vi "FilterPointNameToFloat.vi"(11 "RobotPoints in":string[][](array[string])) -> (0 "U":dbl, 1 "Z":dbl, 2 "V":dbl, 3 "Hand":string, 4 "Y":dbl, 5 "W":dbl, 6 "X":dbl)   [LabVIEW 2019]
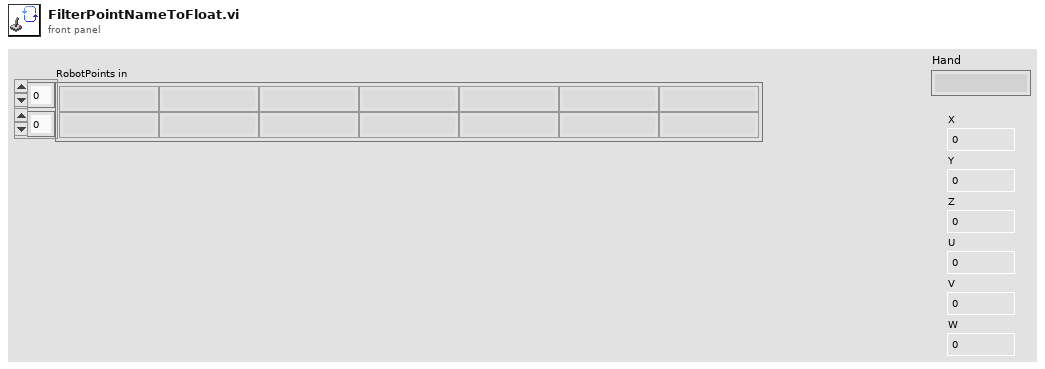
[diagram p1: front panel]
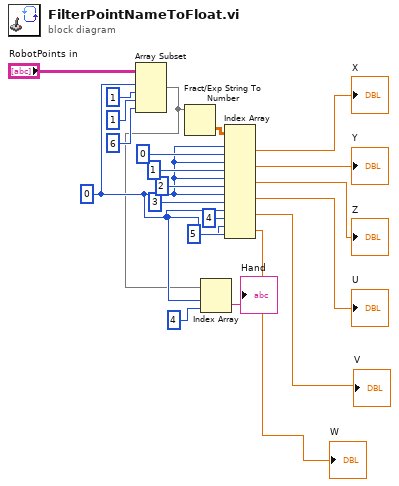
[diagram p0: block diagram]
diagram:
  w4 = 0 ("index")
  n1 = Array Subset(array="RobotPoints in", index (row)=w4, length (row)=1 ("length"), index (col)=1 ("index"), length (col)=6 ("length")) -> (w3:string[][])
  n2 = Fract/Exp String To Number(string=w3) -> (number=w5:dbl[][])  [unwired: 3 in, 1 out]
  n3 = Index Array(array=w3, index (row)=w4, index (col)=4 ("disabled index (col)")) -> (element=→"Hand":string)
  n4 = Index Array(array=w5, index (row) #1=w4, index (col) #1=0 ("disabled index (col)"), index (row) #2=w4, index (col) #2=1 ("disabled index (col)"), index (row) #3=w4, index (col) #3=2 ("disabled index (col)"), index (row) #4=w4, index (col) #4=3 ("disabled index (col)"), index (row) #5=w4, index (col) #5=4 ("disabled index (col)"), index (row) #6=w4, index (col) #6=5 ("disabled index (col)")) -> (element #1=→"X":dbl, element #2=→"Y":dbl, element #3=→"Z":dbl, element #4=→"U":dbl, element #5=→"V":dbl, element #6=→"W":dbl)
